vi "Robot Systems.vi"(11 "input cluster":T1) -> ()   [LabVIEW 2015]
uses:
  Joystick/ControlsToCommands.ctl
  Robot Global Data.vi
panel:
  in  "Speed":dbl
  in  "Time":dbl
  out "Output":bool
  out "What to do":string
  out "Temporary Center":dbl
  out "Stuck?":bool
  out "Position":dbl
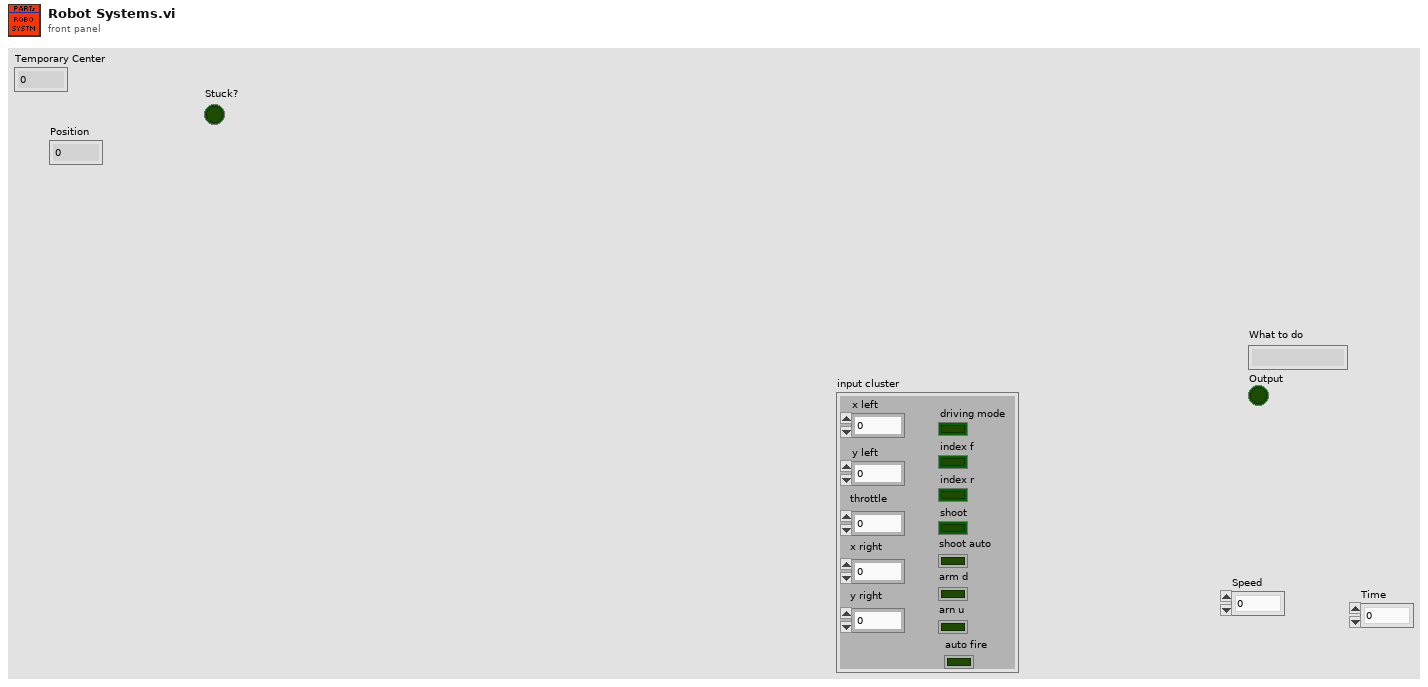
[diagram p1: front panel]
types:
  T1 = typedef "ControlsToCommands.ctl" = cluster{"x left":dbl, "y left":dbl, "throttle":dbl, "x right":dbl, "y right":dbl, "driving mode":bool, "index f":bool, "index r":bool, "shoot":bool, "shoot auto":bool, "arm d":bool, "arn u":bool, "auto fire":bool}
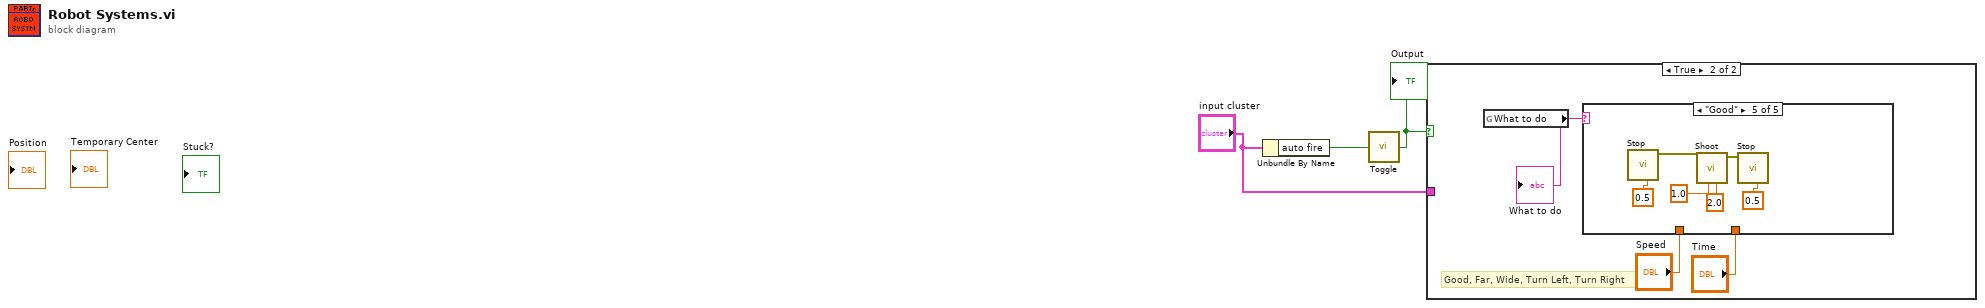
[diagram p0: block diagram]
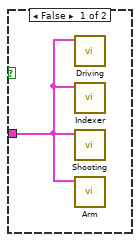
[diagram p2: hidden frame]
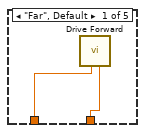
[diagram p3: hidden frame]
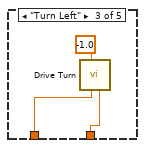
[diagram p5: hidden frame]
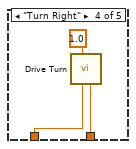
[diagram p6: hidden frame]
diagram:
  n1 = Unbundle By Name("input cluster") -> ("auto fire"=w2:bool)
  n2 = call "Toggle.vi"("Input"=w2) -> ("Output"=w1:bool)  [unwired: 4 in]
  "Output" <- w1
  n3 = case shown="True" w1 {
    tunnel: "input cluster" -> [w4 _]
    frame False {
      n4 = call "Driving.vi"("input cluster"=w4) -> ()  [unwired: 11 in]
      n5 = call "Indexer.vi"("input cluster"=w4) -> ()  [unwired: 11 in]
      n6 = call "Shooting.vi"("input cluster"=w4) -> ()  [unwired: 11 in]
      n7 = call "Arm.vi"("input cluster"=w4) -> ()  [unwired: 11 in]
    }
    frame True {
      # "Good, Far, Wide, Turn Left, Turn Right"
      n8 = global read "Robot Global Data.vi" "What to do"() -> (w7:string)
      "What to do" <- w7
      n9 = case shown="\"Good\"" w7 {
        tunnel: "Time" -> [w9 _ w11 w14 _]
        tunnel: "Speed" -> [w8 _ w10 w13 _]
        frame "Far", Default {
          n10 = call "Drive Forward.vi"("Time"=w9, "Speed"=w8) -> ()  [unwired: 9 in, 1 out]
        }
        frame "Wide" {
        }
        frame "Turn Left" {
          n11 = call "Drive Turn.vi"("Time"=w11, "Speed"=w10, "Direction"=-1.0) -> ()  [unwired: 8 in, 1 out]
        }
        frame "Turn Right" {
          n12 = call "Drive Turn.vi"("Time"=w14, "Speed"=w13, "Direction"=1.0) -> ()  [unwired: 8 in, 1 out]
        }
        frame "Good" {
          n13 = call "Stop.vi"("Time"=0.5) -> ("error out"=w16:errorcluster)  [unwired: 10 in]
          n14 = call "Shoot.vi"("Time"=2.0, "Speed"=1.0, "error in"=w16) -> ("error out"=w19:errorcluster)  [unwired: 8 in]
          n15 = call "Stop.vi"("Time"=0.5, "error in"=w19) -> ()  [unwired: 9 in, 1 out]
        }
      }
    }
  }
